vi "svl_Equivalent Continuous Level (1 Ch).vi"(8 "error in (no error)":errorcluster, 9 "processing state":T1(ring), 11 "scaledSignal":waveform(dbl)={"t0"=timestamp(0 s since 1904-01-01), "dt"=0.0, "Y"=[]}) -> (0 "error out":errorcluster, 3 "equivalent continuous level [EU^2 rms]":dbl format="%.2f")   [LabVIEW 2017]
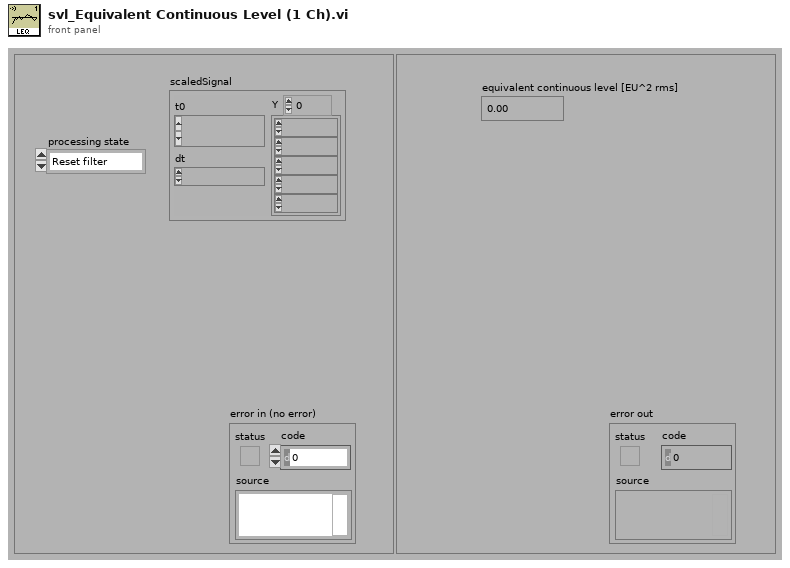
[diagram p1: front panel]
types:
  T1 = enum16{"Reset filter", "Restart averaging", "Continue processing"}
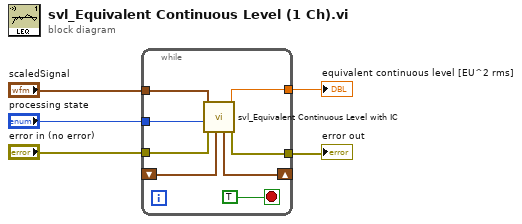
[diagram p0: block diagram]
diagram:
  n1 = while {
    tunnel: [w12] -> w5
    shift-left: _ -> [w10]
    shift-right: [w11] -> _
    tunnel: [w8] -> w4
    tunnel: "error in (no error)" -> [w9]
    tunnel: "processing state" -> [w7]
    tunnel: "scaledSignal" -> [w6]
    stop <- TRUE stop-if-true
    n2 = call <vilib>:"svl_Equivalent Continuous Level with IC.vi"("state in"=w10, "error in (no error)"=w9, "processing state"=w7, "scaledSignal"=w6) -> ("error out"=w8:errorcluster, "Numeric"=w12:dbl, "state out"=w11:cluster{dbl, dbl})  [unwired: 5 in]
  }
  "equivalent continuous level [EU^2 rms]" <- w5
  "error out" <- w4
